vi "enumerateStaticDependencies.vi"(8 "error in (no error)":errorcluster, 11 "Instrument":refnum<class "Instrument.lvclass">) -> (0 "error out":errorcluster, 2 "Static Dependencies":refnum<class "Dependency.lvclass">[](array[class]), 3 "Instrument out":refnum<class "Instrument.lvclass">)   [LabVIEW 2019, in "Instrument.lvlib" / "Instrument.lvclass"]
doc: "JKI State Machine Objects (SMO) 1.3.0.56\nJKI - JKI\nCopyright (c) 2017, JKI"
uses:
  Instrument.lvclass
  C:/Program Files/National Instruments/LabVIEW 2019/vi.lib/JKI/JKI SMO/SMO/SMO.lvclass
  <vilib>/JKI/JKI SMO/Dependency/Dependency.lvclass
  Typedefs/Dependencies--Enum.ctl
  <userlib>/LevyLab/Debug/Attribute.Debug/DebugBehavior.ctl
  Instrument.lvclass/Instrument.ctl
  <userlib>/LevyLab/Logger.Error/Logger.Error/Logger.Error.lvclass/Logger.Error.ctl
  <userlib>/LevyLab/Logger.PGSQL/Logger.PGSQL/Logger.PGSQL.lvclass
  <userlib>/LevyLab/Logger.Error/Logger.Error/Logger.Error.lvclass
  <userlib>/LevyLab/RemoteControl/RemoteControl/RemoteControl.lvclass
  subsystems/HAL/HAL.lvclass
  <vilib>/JKI/JKI SMO/SMO/SMO.lvclass
  <userlib>/LevyLab/Debug/Debug.lvlib
  <userlib>/LevyLab/Debug/Attribute.Debug/Attribute.Debug.lvclass
  C:/Program Files/National Instruments/LabVIEW 2019/user.lib/LevyLab/Logger/Logger/Logger.lvclass
panel:
  # "For instructions on how to use the JKI State Machine Objects, examples and video tutorials, visit:\nhttp://jki.net/state-machine-objects/\n\nJKI State Machine Objects™\nhttp://jki.net/state-machine-objects/\nCopyright (C) 2005-2015, JKI <info@jki.net>\nALL RIGHTS RESERVED"
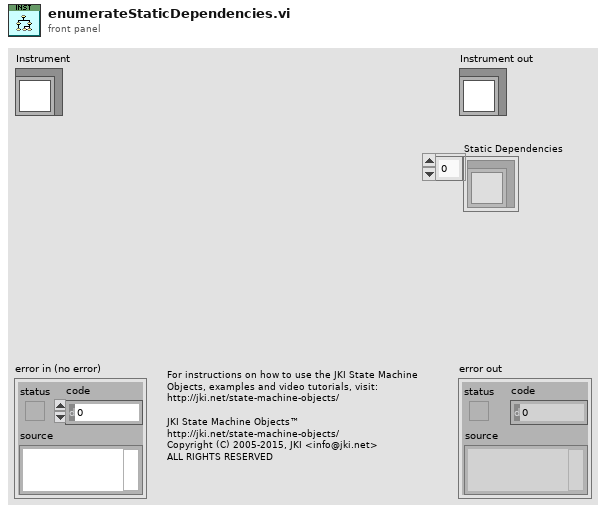
[diagram p1: front panel]
types:
  T1 = typedef "Debug.lvlib/Attribute.Debug.lvclass/DebugBehavior.ctl" = enum16{"Normal", "Debug"}
  T2 = typedef "Instrument.lvlib/Instrument.lvclass/Dependencies--Enum.ctl" = enum16{"API", "Configuration", "HAL", "DB-Logger", "Error-Logger", "Remote-Control"}
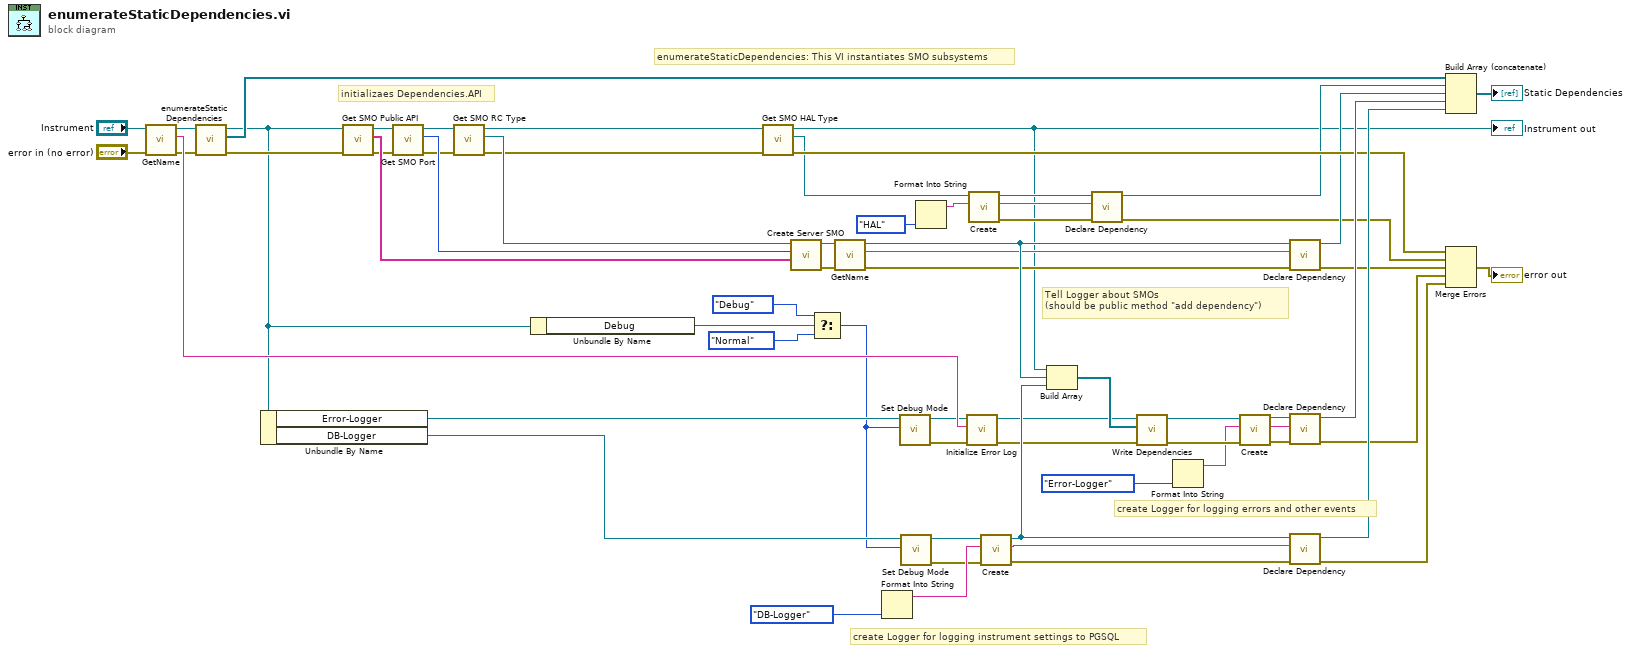
[diagram p0: block diagram]
diagram:
  # "initializaes Dependencies.API"
  # "enumerateStaticDependencies: This VI instantiates SMO subsystems"
  # "Tell Logger about SMOs\n(should be public method \"add dependency\")"
  # "create Logger for logging errors and other events"
  # "create Logger for logging instrument settings to PGSQL"
  n1 = call <vilib>:"GetName.vi"("error in (no error)"="error in (no error)", "SMO"="Instrument") -> ("error out"=w30:errorcluster, "Name"=w41:string, "SMO out"=w62:refnum<class "Instrument.lvclass">)  [unwired: 6 in, 1 out]
  n2 = call-parent "enumerateStaticDependencies.vi"("error in (no error)"=w30, "SMO"=w62) -> ("error out"=w9:errorcluster, "Static Dependencies"=w46:refnum<class "Dependency.lvclass">[], "SMO out"=w5:refnum<class "Instrument.lvclass">)  [unwired: 7 in]
  n3 = Unbundle By Name(w5) -> ("Error-Logger"=w10:refnum<class "Logger.Error.lvclass">, "DB-Logger"=w11:refnum<class "Logger.PGSQL.lvclass">)
  n4 = call-dynamic "Get SMO Public API.vi"("error in (no error)"=w9, "Instrument in"=w5) -> ("error out"=w29:errorcluster, "commands"=w38:string[], "Instrument out"=w55:refnum<class "Instrument.lvclass">)  [unwired: 7 in]
  n5 = call-dynamic "Get SMO Port.vi"("error in (no error)"=w29, "Instrument in"=w55) -> ("error out"=w28:errorcluster, "Port"=w37:u16, "Instrument out"=w40:refnum<class "Instrument.lvclass">)  [unwired: 7 in]
  n6 = call-dynamic "Get SMO RC Type.vi"("error in (no error)"=w28, "Instrument in"=w40) -> ("error out"=w8:errorcluster, "RemoteControl"=w39:refnum<class "RemoteControl.lvclass">, "Instrument out"=w4:refnum<class "Instrument.lvclass">)  [unwired: 7 in]
  n7 = Unbundle By Name(w5) -> ("Debug"=w7:bool)
  n8 = call-dynamic "Get SMO HAL Type.vi"("error in (no error)"=w8, "Instrument in"=w4) -> ("error out"=w31:errorcluster, "Dependencies.HAL"=w19:refnum<class "HAL.lvclass">, "Instrument out"=w1:refnum<class "Instrument.lvclass">)  [unwired: 7 in]
  "Instrument out" <- w1
  n9 = call <userlib>:"Create Server SMO.vi"("Commands"=w38, "Port"=w37, "RemoteControl in"=w39) -> ("error out"=w48:errorcluster, "RemoteControl out"=w49:refnum<class "RemoteControl.lvclass">)  [unwired: 7 in]
  n10 = Select(t=DebugBehavior."Debug" ("Behavior (Normal)"), s=w7, f=DebugBehavior."Normal" ("Behavior (Normal)")) -> (s? t:f=w6:T1)
  n11 = call <vilib>:"GetName.vi"("error in (no error)"=w48, "SMO"=w49) -> ("error out"=w25:errorcluster, "Name"=w26:string, "SMO out"=w27:refnum<class "RemoteControl.lvclass">)  [unwired: 6 in, 1 out]
  n12 = Format Into String(Dependencies--Enum."DB-Logger" ("Dependencies")) -> (resulting string=w32:string)  [unwired: 3 in, 1 out]
  n13 = call <userlib>:"Set Debug Mode.vi"("Behavior"=w6, "SMO"=w10) -> ("error out"=w15:errorcluster, "SMO out"=w12:refnum<class "Logger.Error.lvclass">)  [unwired: 8 in]
  n14 = call <userlib>:"Set Debug Mode.vi"("Behavior"=w6, "SMO"=w11) -> ("error out"=w13:errorcluster, "SMO out"=w14:refnum<class "Logger.PGSQL.lvclass">)  [unwired: 8 in]
  n15 = Format Into String(Dependencies--Enum."HAL" ("Dependencies")) -> (resulting string=w20:string)  [unwired: 3 in, 1 out]
  n16 = call <userlib>:"Initialize Error Log.vi"("error in (no error)"=w15, "Application Name"=w41, "Logger.Error in"=w12) -> ("error out"=w42:errorcluster, "Logger.Error out"=w43:refnum<class "Logger.Error.lvclass">)  [unwired: 7 in]
  n17 = call <vilib>:"Create.vi"("Subsystem Name (optional)"=w20, "SMO"=w19) -> ("error out"=w16:errorcluster, "SMO name"=w18:string, "SMO out"=w17:refnum<class "HAL.lvclass">)  [unwired: 7 in]
  n18 = call <vilib>:"Create.vi"("error in (no error)"=w13, "Subsystem Name (optional)"=w32, "SMO"=w14) -> ("error out"=w57:errorcluster, "SMO name"=w44:string, "SMO out"=w51:refnum<class "Logger.PGSQL.lvclass">)  [unwired: 6 in]
  n19 = Build Array(w1, w27, w51) -> (w50:refnum<class "SMO.lvclass">[])
  n20 = call <vilib>:"Declare Dependency.vi"("error in (no error)"=w16, "Name"=w18, "Type"=w17) -> ("error out"=w22:errorcluster, "Dependency out"=w21:refnum<class "Dependency.lvclass">)  [unwired: 7 in]
  n21 = call <userlib>:"Write Dependencies.vi"("error in (no error)"=w42, "SMOs"=w50, "Logger.Error in"=w43) -> ("error out"=w52:errorcluster, "Logger.Error out"=w53:refnum<class "Logger.Error.lvclass">)  [unwired: 7 in]
  n22 = Format Into String(Dependencies--Enum."Error-Logger" ("Dependencies")) -> (resulting string=w34:string)  [unwired: 3 in, 1 out]
  n23 = call <vilib>:"Create.vi"("error in (no error)"=w52, "Subsystem Name (optional)"=w34, "SMO"=w53) -> ("error out"=w58:errorcluster, "SMO name"=w45:string, "SMO out"=w59:refnum<class "Logger.Error.lvclass">)  [unwired: 6 in]
  n24 = call <vilib>:"Declare Dependency.vi"("error in (no error)"=w25, "Name"=w26, "Type"=w27) -> ("error out"=w24:errorcluster, "Dependency out"=w23:refnum<class "Dependency.lvclass">)  [unwired: 7 in]
  n25 = call <vilib>:"Declare Dependency.vi"("error in (no error)"=w58, "Name"=w45, "Type"=w59) -> ("error out"=w47:errorcluster, "Dependency out"=w60:refnum<class "Dependency.lvclass">)  [unwired: 7 in]
  n26 = call <vilib>:"Declare Dependency.vi"("error in (no error)"=w57, "Name"=w44, "Type"=w51) -> ("error out"=w54:errorcluster, "Dependency out"=w56:refnum<class "Dependency.lvclass">)  [unwired: 7 in]
  n27 = Build Array (concatenate)(w46, w21, w23, w60, w56) -> (→"Static Dependencies":refnum<class "Dependency.lvclass">[])
  n28 = Merge Errors(w31, w22, w24, w47, w54) -> (→"error out":errorcluster)
